vi "setVoltageOn.vi"(9 "Mode":bool, 10 "Current Temperature (Simulated)":refnum<vi>, 11 "Room Temperature (K)":refnum<vi>) -> (3 "Value":dbl)   [LabVIEW 2013]
uses:
  Controls/FGV Function.ctl
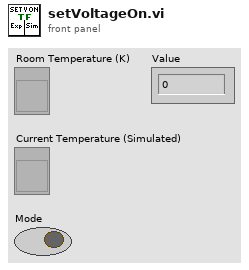
[diagram p1: front panel]
types:
  T1 = typedef "FGV Function.ctl" = enum16{"Initiate", "Read", "Set On", "Set Off"}
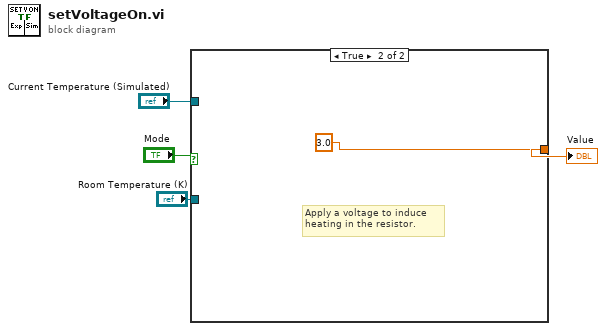
[diagram p0: block diagram]
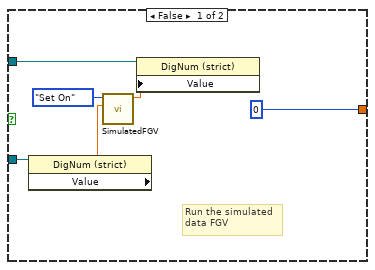
[diagram p2: hidden frame]
diagram:
  n1 = case shown="True" "Mode" {
    tunnel: [0 3.0 ("data")] -> w4
    tunnel: "Room Temperature (K)" -> [w6 _]
    tunnel: "Current Temperature (Simulated)" -> [w5 _]
    frame False {
      # "Run the simulated\ndata FGV"
      n2 = property on="Property Node" class="DigNum (strict)"(reference=w6) -> ("Value"=w10:dbl)  [unwired: 1 in, 2 out]
      n3 = call "SimulatedFGV.vi"("Starting Temperature"=w10, "FGV Function"=FGV_Function."Set On") -> ("Current Temperature"=w7:dbl)  [unwired: 9 in]
      n4 = property on="Property Node" class="DigNum (strict)"(reference=w5, "Value"=w7) -> ()  [unwired: 1 in, 2 out]
    }
    frame True {
      # "Apply a voltage to induce \nheating in the resistor."
    }
  }
  "Value" <- w4
